vi "FITS_Read_Header.vi"(5 "Path":path, 6 "Load ?":bool, 7 "FITS in":string) -> (0 "error out":errorcluster, 1 "Header":T1={"Naxis"=0, "Naxis1"=0, "Naxis2"=0, "Naxis3"=0, "DataType"=32, "Bscale"=0.0, "Bzero"=0.0} {"DataType" items=["U8"=8, "I16"=16, "I32"=32, "SGL (float)"=-32, "DBL"=-64]}, 2 "FITS data":string, 3 "FITS header":string)   [LabVIEW 2020]
doc: "This vi allows to save images of SGL data into FITS format. The input data may indifferently be a single image or a cube of images. In any case, the data have to be converted into a 1-D array. The dimensions of the data cube must, however, be provided in input : they are naxis1, naxis2, naxis3. For a single image, set naxis3 to 1 (or any integer value less or equal to 1)."
panel:
  out "Naxis":i32
  out "Naxis_Found":bool
  out "Naxis1":i32
  out "Naxis1_Found":bool
  out "Naxis2":i32
  out "Naxis2_Found":bool
  out "Naxis3":i32
  out "Naxis3_Found":bool
  out "Bitpix":i32
  out "Bitpix_Found":bool
  out "Bscale":dbl
  out "Bscale_Found":bool
  out "Bzero":dbl
  out "Bzero_Found":bool
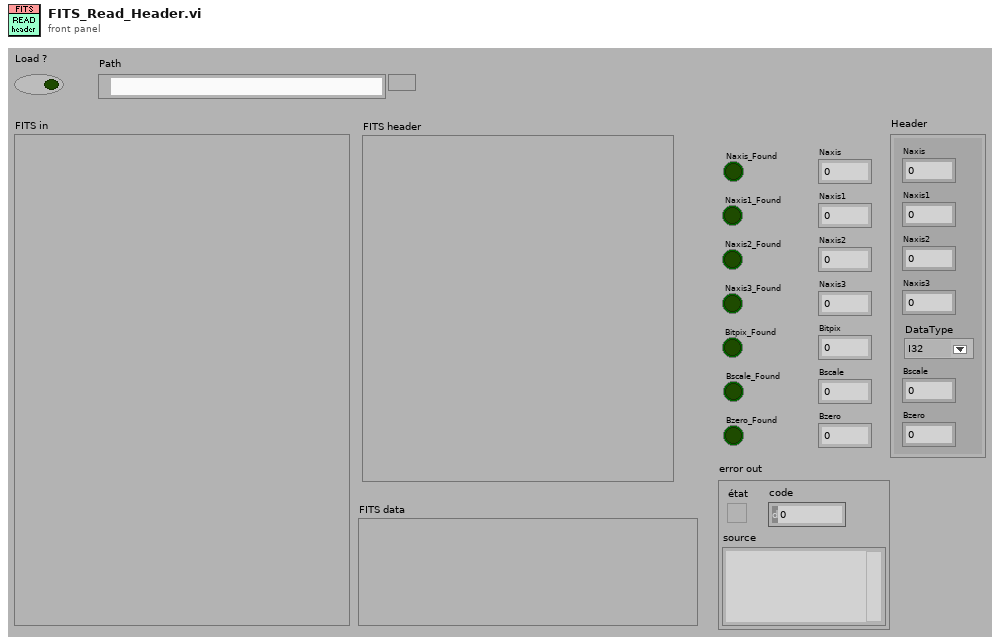
[diagram p1: front panel]
types:
  T1 = cluster{"Naxis":i32, "Naxis1":i32, "Naxis2":i32, "Naxis3":i32, "DataType":i32, "Bscale":dbl, "Bzero":dbl}
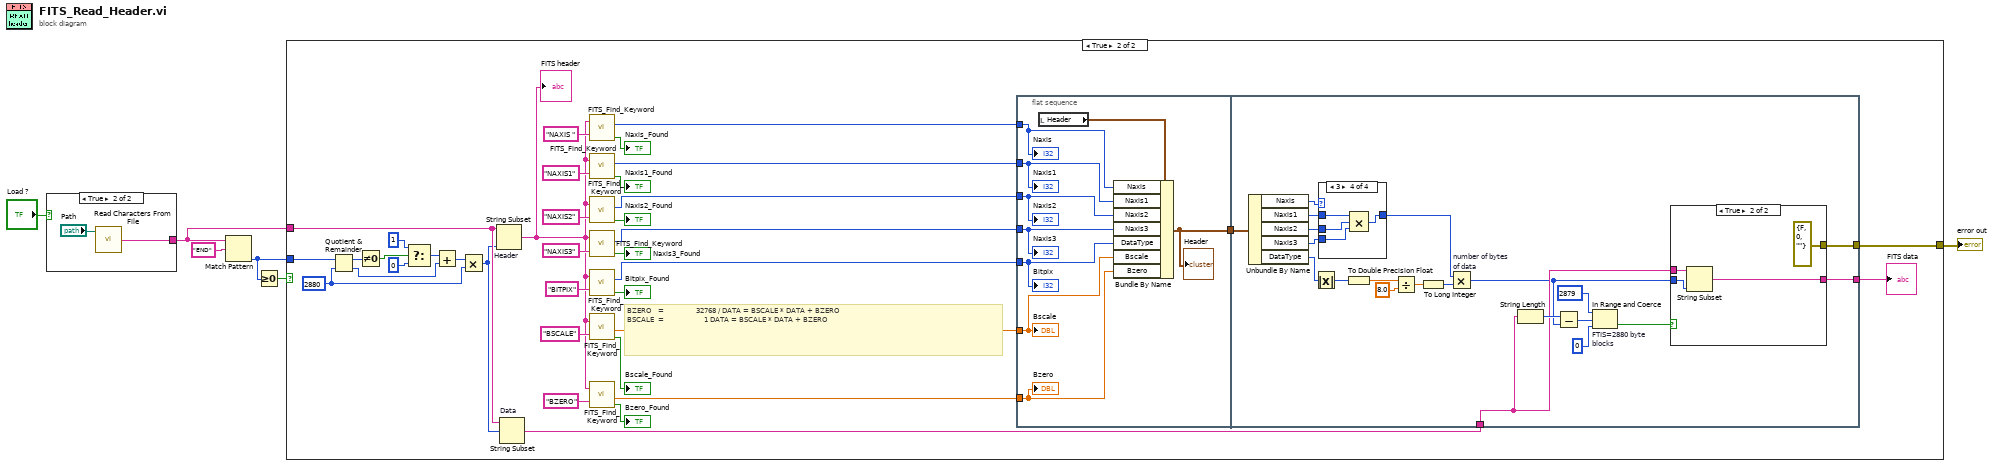
[diagram p0: block diagram]
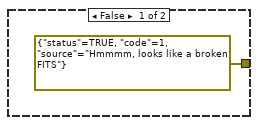
[diagram p2: hidden frame]
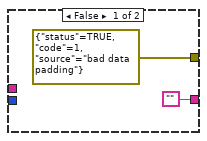
[diagram p3: hidden frame]
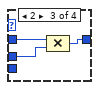
[diagram p6: hidden frame]
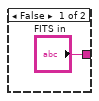
[diagram p7: hidden frame]
diagram:
  n1 = case shown="True" "Load ?" {
    tunnel: ["FITS in" w8] -> w4
    frame False {
    }
    frame True {
      n2 = call <vilib>:"Read Characters From File.vi"("file path (dialog if empty)"="Path") -> ("character string"=w8:string)  [unwired: 5 in, 3 out]
    }
  }
  n3 = Match Pattern(string=w4, regular expression="END") -> (offset past match=w2:i32)  [unwired: 1 in, 3 out]
  n4 = Greater Or Equal To 0?(x=w2) -> (x >= 0?=w1:bool)
  n5 = case shown="True" w1 {
    tunnel: w4 -> [_ w41]
    tunnel: [errorcluster {"status"=TRUE, "code"=1, "source"="Hmmmm, looks like a broken FITS"} ("error out") w36] -> w3
    tunnel: w2 -> [_ w35]
    frame False {
    }
    frame True {
      w42 = 2880
      # "BZERO   =                32768 / DATA = BSCALE * DATA + BZERO                  \nBSCALE  =                    1 DATA = BSCALE * DATA + BZERO"
      n6 = Quotient & Remainder(x=w35, y=w42) -> (x-y*floor(x/y)=w39:i32, floor(x/y)=w37:i32)
      n7 = Not Equal To 0?(x=w39) -> (x != 0?=w46:bool)
      n8 = Select(t=1, s=w46, f=0) -> (s? t:f=w38:i32)
      n9 = Add(x=w38, y=w37) -> (x+y=w43:i32)
      n10 = Multiply(x=w43, y=w42) -> (x*y=w40:i32)
      n11 = String Subset "Header"(string=w41, length (rest)=w40) -> (substring=w18:string)  [unwired: 1 in]
      "FITS header" <- w18
      n12 = String Subset "Data"(string=w41, offset (0)=w40) -> (substring=w34:string)  [unwired: 1 in]
      n13 = call "FITS_Find_Keyword.vi"("FITS bytes"=w18, "Keyword"="NAXIS ") -> ("I32 value"=w14:i32, "Found ?"=→"Naxis_Found":bool)  [unwired: 2 out]
      n14 = call "FITS_Find_Keyword.vi"("FITS bytes"=w18, "Keyword"="NAXIS1") -> ("I32 value"=w13:i32, "Found ?"=→"Naxis1_Found":bool)  [unwired: 2 out]
      n15 = call "FITS_Find_Keyword.vi"("FITS bytes"=w18, "Keyword"="NAXIS2") -> ("I32 value"=w15:i32, "Found ?"=→"Naxis2_Found":bool)  [unwired: 2 out]
      n16 = call "FITS_Find_Keyword.vi"("FITS bytes"=w18, "Keyword"="NAXIS3") -> ("I32 value"=w16:i32, "Found ?"=→"Naxis3_Found":bool)  [unwired: 2 out]
      n17 = call "FITS_Find_Keyword.vi"("FITS bytes"=w18, "Keyword"="BITPIX") -> ("I32 value"=w17:i32, "Found ?"=→"Bitpix_Found":bool)  [unwired: 2 out]
      n18 = call "FITS_Find_Keyword.vi"("FITS bytes"=w18, "Keyword"="BSCALE") -> ("DBL value"=w11:dbl, "Found ?"=→"Bscale_Found":bool)  [unwired: 2 out]
      n19 = call "FITS_Find_Keyword.vi"("FITS bytes"=w18, "Keyword"="BZERO") -> ("DBL value"=w12:dbl, "Found ?"=→"Bzero_Found":bool)  [unwired: 2 out]
      n20 = flat-sequence {
        tunnel: [w55] -> w47
        tunnel: w14 -> [w52]
        tunnel: w13 -> [w51]
        tunnel: w11 -> [w53]
        tunnel: w12 -> [w54]
        tunnel: w17 -> [w50]
        tunnel: w16 -> [w49]
        tunnel: w15 -> [w48]
        tunnel: w47 -> [w77]
        tunnel: [w66] -> w36
        tunnel: w34 -> [w59]
        tunnel: [w57] -> w33
        frame #0 {
          n21 = local read "Header"() -> (w56:T1)
          n22 = Bundle By Name(cluster=w56, "Naxis"=w52, "Naxis1"=w51, "Naxis2"=w48, "Naxis3"=w49, "DataType"=w50, "Bscale"=w53, "Bzero"=w54) -> (w55:T1)
          "Header" <- w55
          "Naxis" <- w52
          "Naxis1" <- w51
          "Bscale" <- w53
          "Bzero" <- w54
          "Bitpix" <- w50
          "Naxis3" <- w49
          "Naxis2" <- w48
        }
        frame #1 {
          n23 = Unbundle By Name(w77) -> ("Naxis"=w60:i32, "Naxis1"=w76:i32, "Naxis2"=w75:i32, "Naxis3"=w74:i32, "DataType"=w73:i32)
          n24 = Absolute Value(x=w73) -> (abs(x)=w72:i32)
          n25 = case shown="3" w60 {
            selector: w60 -> [w84 _ _ _]
            tunnel: w76 -> [_ w85 w88 w92]
            tunnel: w75 -> [_ _ w87 w91]
            tunnel: w74 -> [_ _ _ w90]
            tunnel: [w84 w85 w86 w89] -> w70
            frame 0, Default {
            }
            frame 1 {
            }
            frame 2 {
              n26 = Compound Arithmetic op=MULTIPLY(w88, w87) -> (w86:i32)
            }
            frame 3 {
              n27 = Compound Arithmetic op=MULTIPLY(w92, w91, w90) -> (w89:i32)
            }
          }
          n28 = To Double Precision Float(number=w72) -> (double precision float=w68:dbl)
          n29 = Divide(x=w68, y=8.0) -> (x/y=w69:dbl)
          n30 = To Long Integer(number=w69) -> (32bit integer=w67:i32)
          n31 = Multiply "number of bytes\nof data"(x=w70, y=w67) -> (x*y=w58:i32)
          n32 = String Length(string=w59) -> (length=w65:i32)
          n33 = Subtract(x=w65, y=w58) -> (x-y=w64:i32)
          n34 = In Range and Coerce "FTIS=2880 byte\nblocks"(upper limit=2879 ("limite haute"), x=w64, lower limit=0 ("limite basse")) -> (In Range?=w61:bool)  [unwired: 1 out]
          n35 = case shown="True" w61 {
            tunnel: [errorcluster {"status"=TRUE, "code"=1, "source"="bad data padding"} ("error out") errorcluster {"status"=FALSE, "code"=0, "source"=""} ("error out")] -> w66
            tunnel: w59 -> [_ w82]
            tunnel: w58 -> [_ w81]
            tunnel: ["" w80] -> w57
            frame False {
            }
            frame True {
              n36 = String Subset(string=w82, length (rest)=w81) -> (substring=w80:string)  [unwired: 1 in]
            }
          }
        }
      }
      "FITS data" <- w33
    }
  }
  "error out" <- w3
